vi "IV-Tracer_v1.02.vi"() -> ()   [LabVIEW 2014]
doc: "Configures a sweep and takes voltage and current readings at each point."
uses:
  <vilib>/Analysis/baseanly.llb/Mean (DBL).vi
  <instrlib>/Keithley 24XX/Public/Data/Read (Multiple Points).vi
  <vilib>/MakerHub/LINX/Public/Peripherals/Analog/Analog Read 1 Chan.vi
  <instrlib>/Keithley 24XX/Keithley 24XX.lvlib
  <instrlib>/Tektronix TDS 200 1000 2000 Series/Tektronix TDS 200 1000 2000 Series.lvlib
  <vilib>/Analysis/NI_AALBase.lvlib
  <vilib>/MakerHub/LINX/LMH-LINX.lvlib
panel:
  in  "Stop Button":bool
  in  "AI Channel":u8
  in  "Serial Port":refnum<visa-resource-name>
  out "Data A0-CH1":string
  in  "File Path Oscillscope":path=path "c:/myfile.txt"
  out "A0 Arduino-CH1 Osc":cluster{"Y":dbl[], dbl[]}(graph)
  in  "Oscilloscope CH1 Probe Attenuation (0.1)":dbl=10.0
  in  "Oscilloscope Source (0: Channel 1)":u16(ring) items=["Channel 1", "Channel 2", "Channel 3", "Channel 4", "Math", "Reference A", "Reference B", "Reference C", "Reference D"]
  in  "Serial Configuration Oscilloscope":T1={"Baud Rate"=9600, "Parity"=0, "Stop Bits"=10, "Flow Control"=2} {"Flow Control" items=["None", "XON/XOFF", "RTS/CTS", "XON/XOFF & RTS/CTS", "DTR/DSR", "XON/XOFF & DTR/DSR"]; "Stop Bits" items=["1.0"=10, "1.5"=15, "2.0"=20]; "Parity" items=["None", "Odd", "Even", "Mark", "Space"]; "Baud Rate" items=["300"=300, "600"=600, "1200"=1200, "2400"=2400, "4800"=4800, "9600"=9600, "19200"=19200]}
  in  "Oscilloscope CH1 Timeout (10000 ms)":u32=10000
  in  "Oscilloscope VISA":refnum<visa-resource-name>
  out "Loop Rate (Hz)":u32
  out "Resistance-Time":sgl[](graph)
  out "spreadsheet string":string
  in  "File Path":path=path "c:/myfile.txt"
  out "IV Curve":cluster{"Voltage":sgl[], "Current":sgl[]}(graph)
  in  "Source Mode  (0: Voltage)":u16(ring) items=["Voltage", "Current"]
  in  "Serial Configuration":T2={"Baud Rate"=9600, "Parity"=0, "Data Bits"=8, "Stop Bits"=10, "Flow Control"=0} {"Flow Control" items=["None", "XON/XOFF", "RTS/CTS", "XON/XOFF & RTS/CTS", "DTR/DSR", "XON/XOFF & DTR/DSR"]; "Stop Bits" items=["1.0"=10, "1.5"=15, "2.0"=20]; "Data Bits" items=["7"=7, "8"=8]; "Parity" items=["None", "Odd", "Even", "Mark", "Space"]; "Baud Rate" items=["300"=300, "600"=600, "1200"=1200, "2400"=2400, "4800"=4800, "9600"=9600, "19200"=19200]}
  in  "VISA resource name":refnum<visa-resource-name>
  in  "Timeout (10000 ms)":i32=10000 format="%#.6g"
  in  "Maximum Amplitude (2)":dbl=2.0
  in  "Minimum Amplitude (1)":dbl=1.0
  in  "Number of Points (5)":u32=5
  in  "Compliance  Level (0.1)":dbl=0.1
  # "(c) 2006 - 2015 National Instruments.  ALL RIGHTS RESERVED."
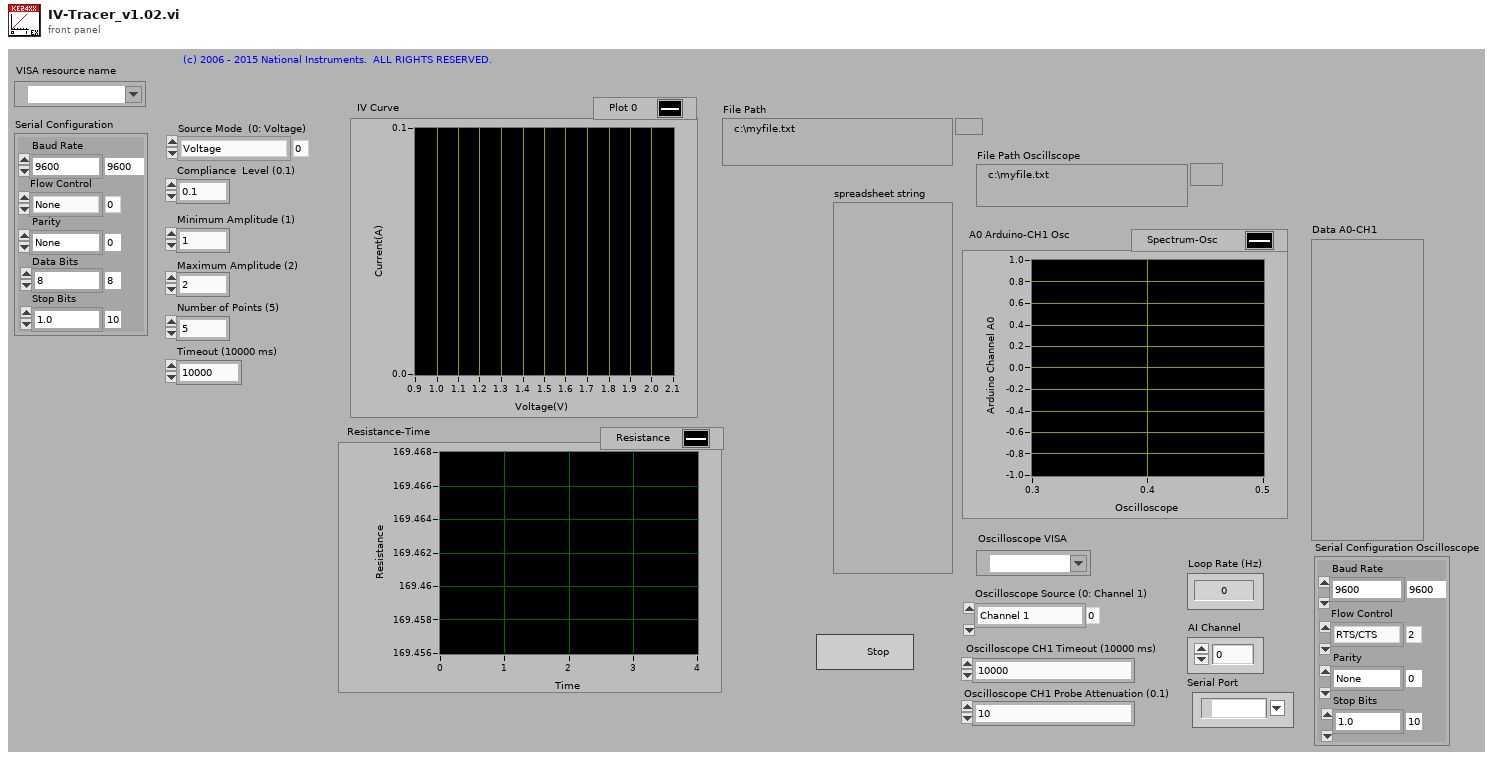
[diagram p1: front panel]
types:
  T1 = cluster{"Baud Rate":u32, "Parity":u16, "Stop Bits":u16, "Flow Control":u16}
  T2 = cluster{"Baud Rate":u32, "Parity":u16, "Data Bits":u16, "Stop Bits":u16, "Flow Control":u16}
  T3 = enum16{"open", "replace", "create", "open or create", "replace or create", "replace or create with confirmation"}
  T4 = typedef "LMH-LINX.lvlib/LINX Ref.ctl" = cluster{"Platform":T5, "Interface":T6, "LINX Device Config":T7}
  T5 = typedef "LMH-LINX.lvlib/Platform.ctl" = enum16{"LINX", "myRIO"}
  T6 = typedef "LMH-LINX.lvlib/Interface.ctl" = enum16{"Serial", "TCP"}
  T7 = typedef "LMH-LINX.lvlib/Device.lvlib/LINX Device Config.ctl" = cluster{"Interface":T6, "COM Port":refnum<visa-resource-name>, "TCP Configuration":T8, "Device Family":u8, "Device ID":u8, "Device Name":string, "TCP Ref":refnum<k5>, "Channels":T9}
  T8 = typedef "LMH-LINX.lvlib/Device.lvlib/TCP Config.ctl" = cluster{"IP Address":string, "Port":u16}
  T9 = typedef "LMH-LINX.lvlib/Channels.ctl" = cluster{"DI":u8[], "DO":u8[], "AI":u8[], "AO":u8[], "PWM":u8[], "QE":u8[], "UART":u8[], "I2C 2":u8[], "SPI":u8[], "CAN":u8[], "Servo":u8[], "AI Ref (V)":dbl, "AO Ref (V)":dbl, "AO Resolution (Bits)":u8}
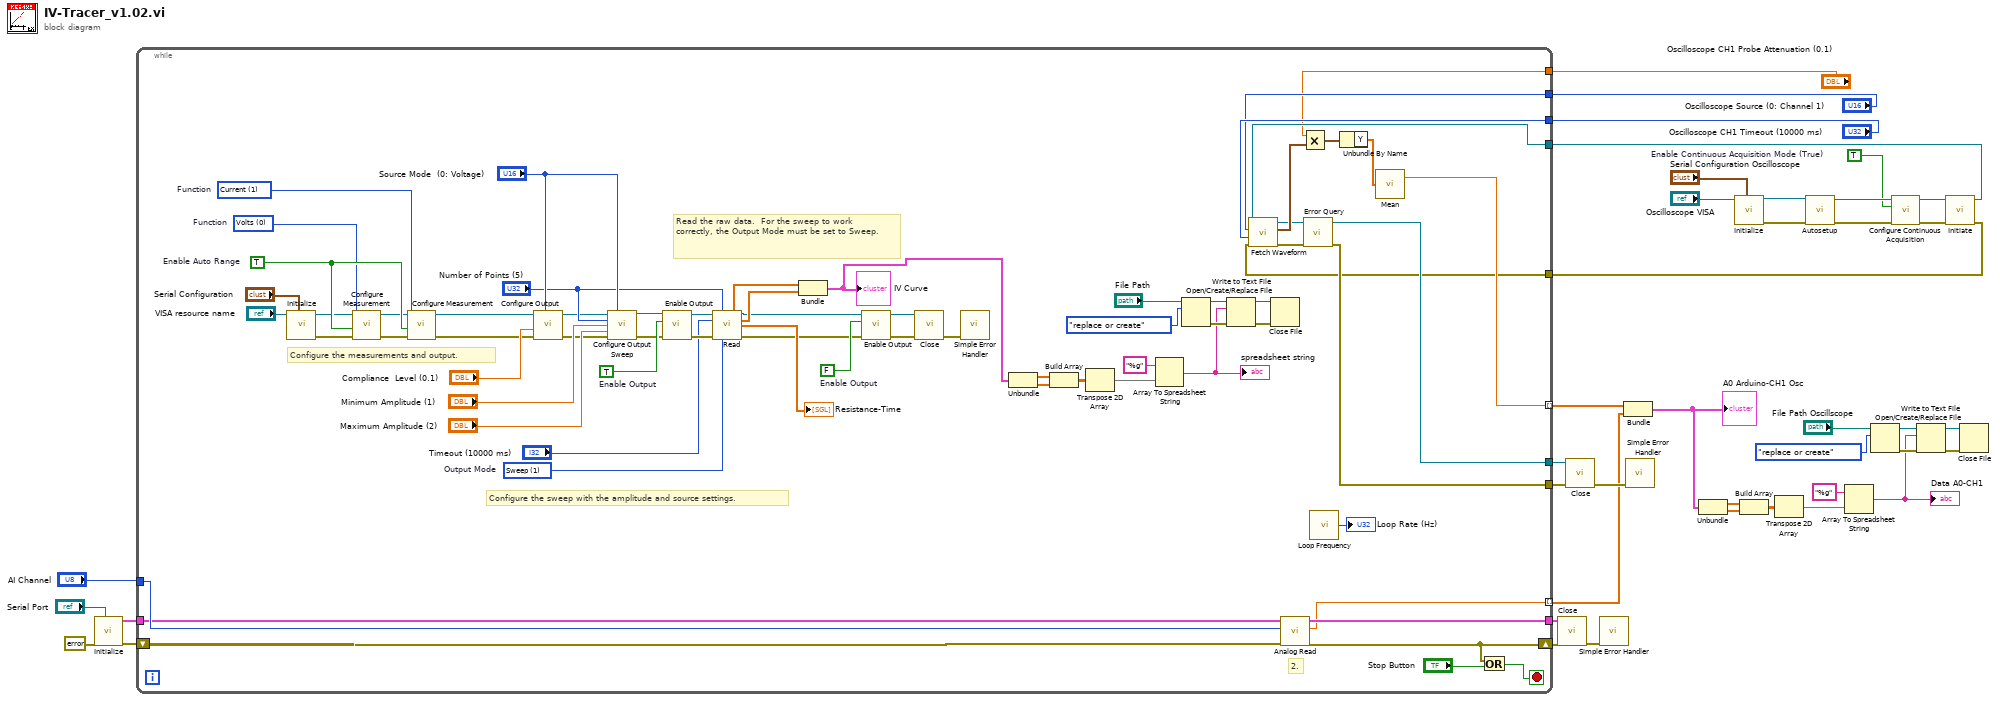
[diagram p0: block diagram]
diagram:
  w34 = TRUE  # Enable Continuous Acquisition Mode (True)
  n1 = call <instrlib>:"Initialize.vi"("Serial Port"="Serial Port", "Error In"=errorcluster {"status"=FALSE, "code"=0, "source"=""}) -> ("Error Out"=w12:errorcluster, "LINX Ref"=w13:T4)  [unwired: 7 in, 1 out]
  n2 = call <instrlib>:"Initialize.vi"("Serial Configuration"="Serial Configuration Oscilloscope", "VISA resource name"="Oscilloscope VISA") -> ("error out"=w39:errorcluster, "VISA resource name out"=w38:refnum<visa-resource-name>)  [unwired: 3 in, 5 out]
  n3 = call <instrlib>:"Autosetup.vi"("error in (no error)"=w39, "VISA resource name"=w38) -> ("error out"=w36:errorcluster, "VISA resource name out"=w35:refnum<visa-resource-name>)  [unwired: 8 out]
  n4 = Open/Create/Replace File(file path (use dialog)="File Path Oscillscope", operation (0:open)=T3."replace or create") -> (refnum out=w25:refnum<file>, error out=w30:errorcluster)  [unwired: 4 in, 1 out]
  n5 = call <instrlib>:"Configure Continuous Acquisition.vi"("error in (no error)"=w36, "Enable Continuous Acquisition Mode (True)"=w34, "VISA resource name"=w35) -> ("error out"=w33:errorcluster, "VISA resource name out"=w32:refnum<visa-resource-name>)  [unwired: 7 out]
  n6 = call <instrlib>:"Initiate.vi"("error in (no error)"=w33, "VISA resource name"=w32) -> ("error out"=w5:errorcluster, "VISA resource name out"=w4:refnum<visa-resource-name>)  [unwired: 8 out]
  n7 = while {
    tunnel: "AI Channel" -> [w103]
    tunnel: w13 -> [w102]
    tunnel: [w100] -> w11
    tunnel: [w99] -> w9 mode=indexing
    tunnel: [w98] -> w8 mode=indexing
    tunnel: [w97] -> w7
    tunnel: [w96] -> w6
    tunnel: w5 -> [w95]
    tunnel: w4 -> [w94]
    tunnel: "Oscilloscope CH1 Timeout (10000 ms)" -> [w93]
    tunnel: "Oscilloscope Source (0: Channel 1)" -> [w92]
    tunnel: "Oscilloscope CH1 Probe Attenuation (0.1)" -> [w91]
    shift-right: [w88] -> w10
    shift-left: w12 -> [w101]
    stop <- w89 stop-if-true
    w70 = TRUE  # Enable Output
    w69 = TRUE  # Enable Auto Range
    w68 = u16 1 items=["Volts", "Current", "Resistance"]  # Function
    w67 = u16 0 items=["Volts", "Current", "Resistance"]  # Function
    w61 = FALSE  # Enable Output
    w55 = u16 1 items=["Fixed", "Sweep", "List"]  # Output Mode
    # "Read the raw data.  For the sweep to work correctly, the Output Mode must be set to Sweep."
    # "Configure the sweep with the amplitude and source settings."
    # "Configure the measurements and output."
    # "2."
    n8 = call <instrlib>:"Initialize.vi"("Serial Configuration"="Serial Configuration", "VISA resource name"="VISA resource name") -> ("error out"=w42:errorcluster, "VISA resource name out"=w41:refnum<visa-resource-name>)  [unwired: 8 in]
    n9 = call <instrlib>:"Configure Measurement.vi"("error in (no error)"=w42, "Enable Auto Range (T:Enable)"=w69, "Function (0: Volts)"=w67, "VISA resource name"=w41) -> ("error out"=w43:errorcluster, "VISA resource name out"=w44:refnum<visa-resource-name>)  [unwired: 6 in]
    n10 = call <instrlib>:"Configure Measurement.vi"("error in (no error)"=w43, "Enable Auto Range (T:Enable)"=w69, "Function (0: Volts)"=w68, "VISA resource name"=w44) -> ("error out"=w46:errorcluster, "VISA resource name out"=w45:refnum<visa-resource-name>)  [unwired: 6 in]
    n11 = call <instrlib>:"Configure Output.vi"("Source Mode  (0: Voltage)"="Source Mode  (0: Voltage)", "error in (no error)"=w46, "Compliance  Level (0.1)"="Compliance  Level (0.1)", "VISA resource name"=w45) -> ("error out"=w47:errorcluster, "VISA resource name out"=w48:refnum<visa-resource-name>)  [unwired: 6 in]
    n12 = call <instrlib>:"Configure Output Sweep.vi"("VISA resource name"=w48, "Source Mode  (0: Voltage)"="Source Mode  (0: Voltage)", "Number of Points (5)"="Number of Points (5)", "Minimum Amplitude (1)"="Minimum Amplitude (1)", "Maximum Amplitude (2)"="Maximum Amplitude (2)", "error in (no error)"=w47) -> ("VISA resource name out"=w64:refnum<visa-resource-name>, "error out"=w65:errorcluster)  [unwired: 8 in]
    n13 = call <instrlib>:"Enable Output.vi"("error in (no error)"=w65, "Enable Output (T: Enable)"=w70, "VISA resource name"=w64) -> ("error out"=w62:errorcluster, "VISA resource name out"=w63:refnum<visa-resource-name>)  [unwired: 7 in]
    n14 = call-poly <instrlib>:"Read.vi"("VISA resource name"=w63, "Sample Count (1)"="Number of Points (5)", "Timeout (10000 ms)"="Timeout (10000 ms)", "error in (no error)"=w62, "Output Mode (0: Fixed)"=w55) -> ("Voltage"=w72:sgl[], "VISA resource name out"=w60:refnum<visa-resource-name>, "Current"=w73:sgl[], "Resistance"=→"Resistance-Time":sgl[], "error out"=w59:errorcluster)  [unwired: 4 in, 2 out]
    n15 = Bundle("Voltage"=w72, "Current"=w73) -> (w86:cluster{"Voltage":sgl[], "Current":sgl[]})  [unwired: 1 out]
    "IV Curve" <- w86
    n16 = call <instrlib>:"Enable Output.vi"("error in (no error)"=w59, "Enable Output (T: Enable)"=w61, "VISA resource name"=w60) -> ("error out"=w58:errorcluster, "VISA resource name out"=w57:refnum<visa-resource-name>)  [unwired: 7 in]
    n17 = call <vilib>:"Close.vi"("error in (no error)"=w58, "VISA resource name"=w57) -> ("error out"=w56:errorcluster)  [unwired: 9 in]
    n18 = call <vilib>:"Simple Error Handler.vi"("error in (no error)"=w56) -> ()  [unwired: 4 in, 5 out]
    n19 = Unbundle(w86) -> ("Voltage"=w79:sgl[], "Current"=w78:sgl[])
    n20 = Build Array(w79, w78) -> (w77:sgl[][])
    n21 = Transpose 2D Array(2D array=w77) -> (transposed array=w75:sgl[][])
    n22 = Array To Spreadsheet String(array=w75, 3:"%g" ("format string")) -> (spreadsheet string=w74:string)  [unwired: 1 in]
    "spreadsheet string" <- w74
    n23 = Open/Create/Replace File(file path (use dialog)="File Path", operation (0:open)=T3."replace or create") -> (refnum out=w80:refnum<file>, error out=w85:errorcluster)  [unwired: 4 in, 1 out]
    n24 = Write to Text File(file (use dialog)=w80, text=w74, error in=w85) -> (refnum out=w83:refnum<file>, error out=w84:errorcluster)  [unwired: 2 out]
    n25 = call <instrlib>:"Fetch Waveform.vi"("error in (no error)"=w95, "Timeout (10000 ms)"=w93, "Source (0: Channel 1)"=w92, "VISA resource name"=w94) -> ("error out"=w106:errorcluster, "Waveform Data"=w108:waveform(dbl), "VISA resource name out"=w105:refnum<visa-resource-name>)  [unwired: 5 out]
    n26 = Close File(refnum=w83, error in=w84) -> ()  [unwired: 2 out]
    n27 = call-poly <vilib>:"Analog Read.vi"("Error In"=w101, "Analog Channel"=w103, "LINX Resource"=w102) -> ("Error Out"=w88:errorcluster, "AI Value"=w99:dbl, "LINX Resource"=w100:T4)  [unwired: 5 in, 1 out]
    n28 = Multiply(x=w91, y=w108) -> (x*y=w107:waveform(dbl))
    n29 = call <instrlib>:"Error Query.vi"("error in (no error)"=w106, "VISA resource name"=w105) -> ("error out"=w96:errorcluster, "VISA resource name out"=w97:refnum<visa-resource-name>)  [unwired: 8 out]
    n30 = call <vilib>:"Loop Frequency.vi"() -> ("Loop Rate (Hz)"=→"Loop Rate (Hz)":u32)
    n31 = Unbundle By Name(w107) -> ("Y"=w109:dbl[])
    n32 = call-poly <vilib>:"Mean.vi"("X"=w109) -> ("mean"=w98:dbl)  [unwired: 1 out]
    n33 = Or(x=w88, y="Stop Button") -> (x .or. y?=w89:bool)
  }
  n34 = call <vilib>:"Close.vi"("Error In"=w10, "LINX Resource"=w11) -> ("Error Out"=w17:errorcluster)  [unwired: 8 in, 1 out]
  n35 = call <vilib>:"Close.vi"("error in (no error)"=w6, "VISA resource name"=w7) -> ("error out"=w31:errorcluster)  [unwired: 9 out]
  n36 = call <vilib>:"Simple Error Handler.vi"("error in (no error)"=w17) -> ()  [unwired: 4 in, 5 out]
  n37 = Bundle(w8, w9) -> (w18:cluster{dbl[], dbl[]})  [unwired: 1 out]
  "A0 Arduino-CH1 Osc" <- w18
  n38 = call <vilib>:"Simple Error Handler.vi"("error in (no error)"=w31) -> ()  [unwired: 1 in, 8 out]
  n39 = Unbundle(w18) -> (w24:dbl[], w23:dbl[])
  n40 = Build Array(w24, w23) -> (w22:dbl[][])
  n41 = Transpose 2D Array(2D array=w22) -> (transposed array=w20:dbl[][])
  n42 = Array To Spreadsheet String(array=w20, 3:"%g" ("format string")) -> (spreadsheet string=w19:string)  [unwired: 1 in]
  "Data A0-CH1" <- w19
  n43 = Write to Text File(file (use dialog)=w25, text=w19, error in=w30) -> (refnum out=w28:refnum<file>, error out=w29:errorcluster)  [unwired: 2 out]
  n44 = Close File(refnum=w28, error in=w29) -> ()  [unwired: 2 out]
